vi "Test.vi"   [LabVIEW 2014]
doc: "This VI is called when test mode begins, and will automatically be terminated when it ends. You can add manual or automatic tests and invoke them from the dashboard."
uses:
  Robot Global Data.vi
types:
  T1 = enum16{"Axis for manual Control of arm", "Axis for manual Control of Claw", "Rotate Claw"}
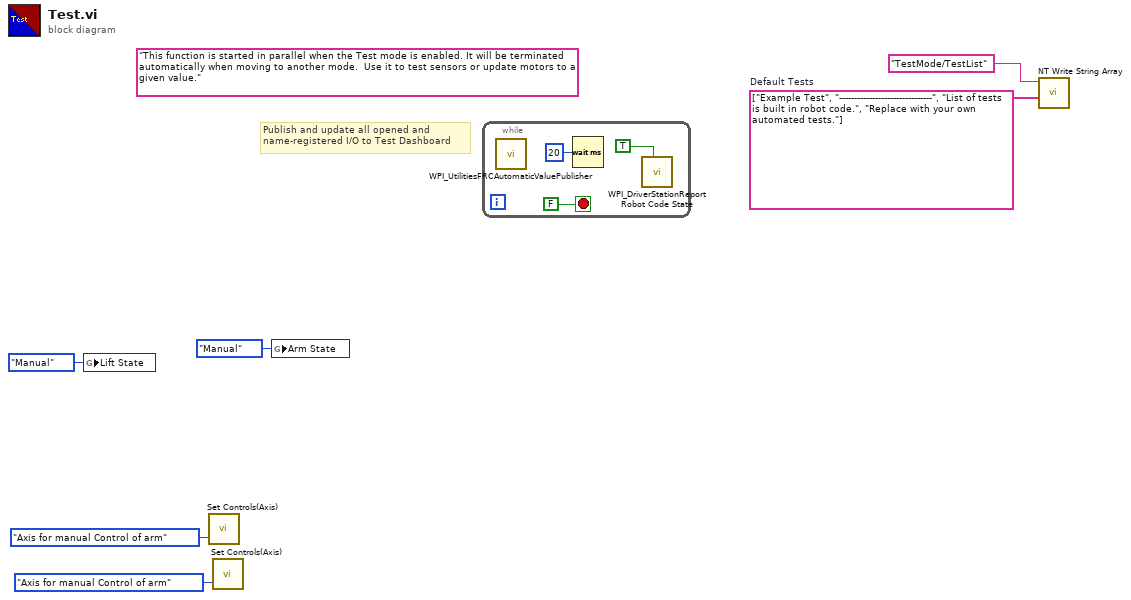
[diagram p0: block diagram]
diagram:
  w6 = string[] ["Example Test", "-------------------------------", "List of tests is built in robot code.", "Replace with your own automated tests."]  # Default Tests
  (unwired) "This function is started in parallel when the Test mode is enabled. It will be terminated automatically when moving to another mode.  Use it to test sensors or update motors to a given value."
  # "Publish and update all opened and\nname-registered I/O to Test Dashboard"
  n1 = global write "Robot Global Data.vi" "Lift State"(enum16{"Initializing", "Running", "Manual"}."Manual" ("Lift State")) -> ()
  n2 = call "Set Controls(Axis).vi"("Axis Actions Secondary"=T1."Axis for manual Control of arm") -> ()  [unwired: 1 in, 2 out]
  n3 = call "Set Controls(Axis).vi"("Axis Actions Secondary"=T1."Axis for manual Control of arm") -> ()  [unwired: 1 in, 2 out]
  n4 = global write "Robot Global Data.vi" "Arm State"(enum16{"Initializing", "Running", "Manual"}."Manual" ("Arm State")) -> ()
  n5 = while {
    stop <- FALSE stop-if-true
    n6 = call <vilib>:"WPI_UtilitiesFRCAutomaticValuePublisher.vi"() -> ()  [unwired: 12 in]
    n7 = Wait (ms)(milliseconds to wait=u32 20) -> ()  [unwired: 1 out]
    n8 = call <vilib>:"WPI_DriverStationReport Robot Code State.vi"("Test"=TRUE ("Autonomous")) -> ()  [unwired: 10 in, 1 out]
  }
  n9 = call <vilib>:"NT Write String Array.vi"("String Array"=w6, "Name"="TestMode/TestList") -> ()  [unwired: 9 in, 1 out]
